vi "Select Model.vi"(10 "SHIFT":enum16{"1", "2", "3", "G"}(ring)) -> (1 "Cancelled":bool, 2 "Initial Data":T2)   [LabVIEW 2017]
uses:
  controls/Model Name.ctl
  GV/All Inputs.vi
panel:
  out "SACB Status":string
  in  "Cancel":bool
  out "Error Out":errorcluster
  out "Connected?":bool caption="Connected to SACB?"
  in  "Model Name":T1=enum."W 501 FRH Std."
  in  "OK Button":bool
  in  "ID":string
  # "Start Autocycle"
  # "Please select the model that you wish to run the autocyle test for, enter the operator ID and then click OK."
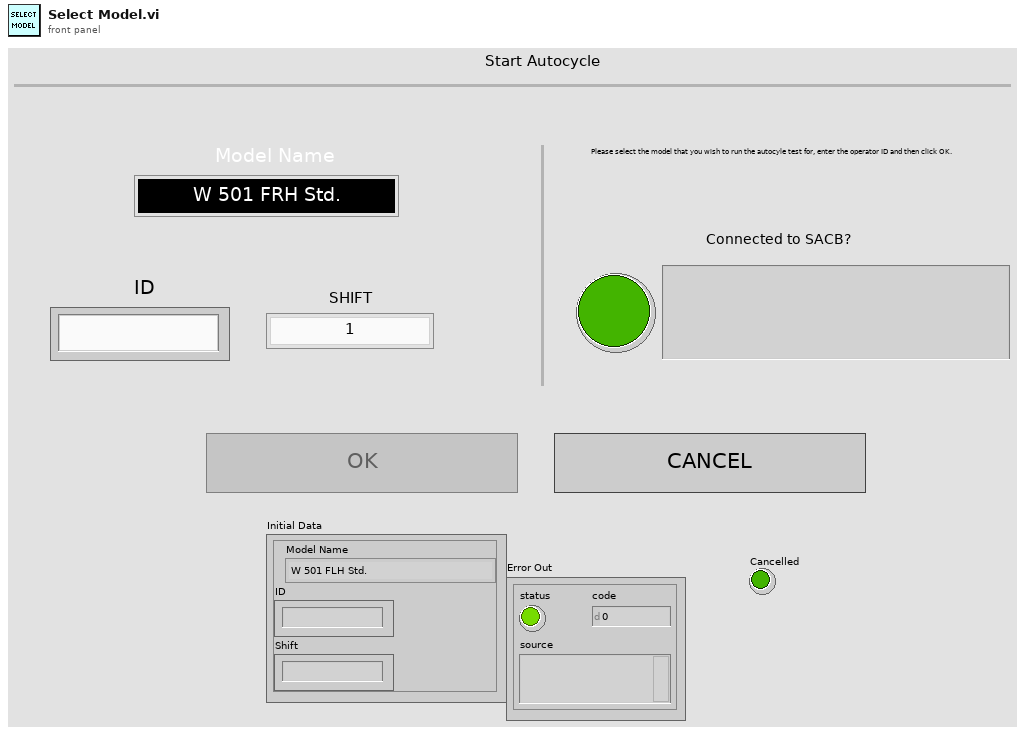
[diagram p1: front panel]
types:
  T1 = typedef "Model Name.ctl" = enum16{"W 501 FLH Std.", "W 501 FRH Std.", "W 601 FR RH Std", "W 601 FR LH Std", "W 601 RR RH Std", "W 601 RR LH Std", "W 601 FR RH AP", "W 601 FR LH AP", "W 601 RR RH AP", "W 601 RR LH AP"}
  T2 = cluster{"Model Name":T1, "ID":string, "Shift":string}
  T3 = enum8{"Enabled", "Disabled", "Disabled and Grayed Out"}
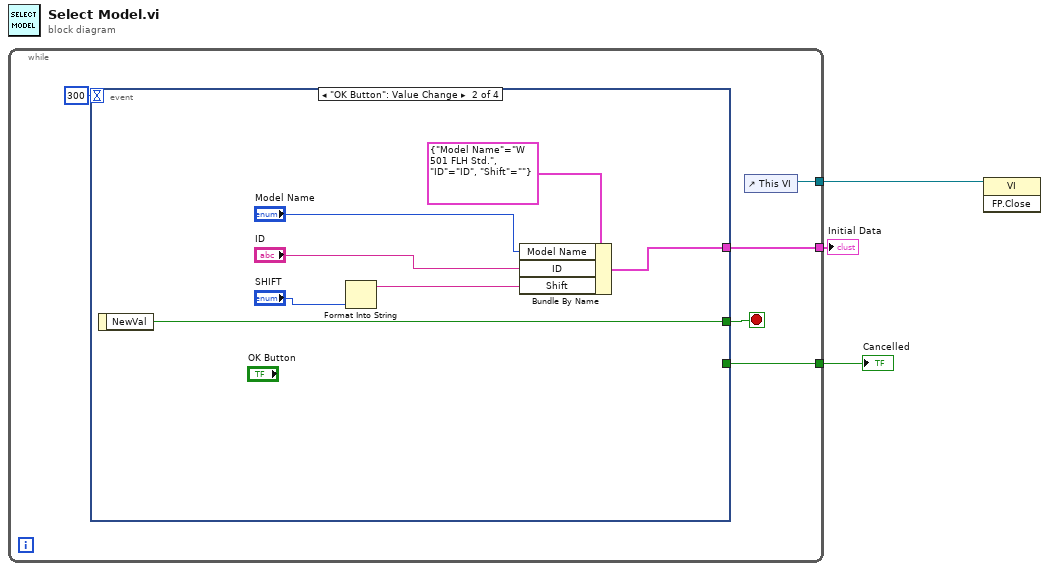
[diagram p0: block diagram]
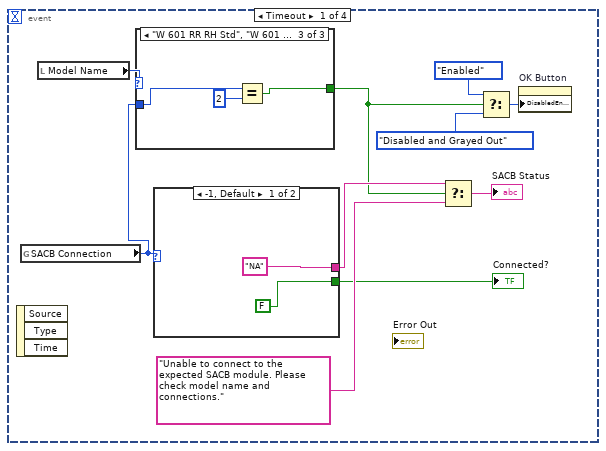
[diagram p2: hidden frame]
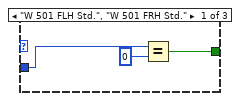
[diagram p3: hidden frame]
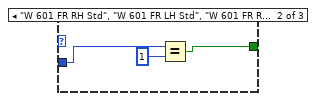
[diagram p4: hidden frame]
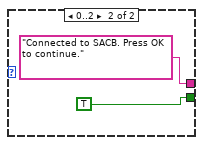
[diagram p5: hidden frame]
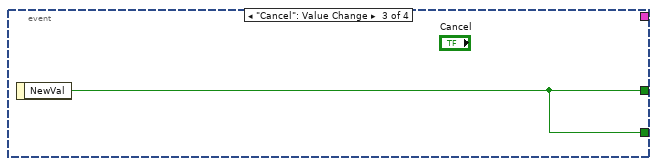
[diagram p6: hidden frame]
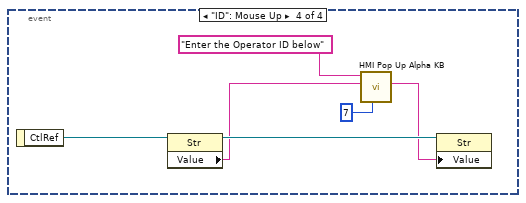
[diagram p7: hidden frame]
diagram:
  n1 = while {
    tunnel: [w8] -> w2
    tunnel: [w5] -> w3
    tunnel: [w4] -> w1
    stop <- w7 stop-if-true
    n2 = event shown="[1] \"OK Button\": Value Change" {
      selector: _ -> [_ _ _ _]
      dyn-events: _ -> [_ _ _ _]
      timeout: 300 -> [_ _ _ _]
      tunnel: [_ w36 _ _] -> w8
      tunnel: [_ w35 w39 _] -> w7
      tunnel: [_ _ w39 _] -> w5
      event Timeout {
        n3 = event-data() -> ()  [unwired: 1 in, 3 out]
        n4 = global read "All Inputs.vi" "SACB Connection"() -> (w10:i32)
        n5 = local read "Model Name"() -> (w11:T1)
        n6 = case shown="\"W 601 RR RH Std\", \"W 601 RR LH Std\", \"W 601 RR RH AP\", \"W 601 RR LH AP\"" w11 {
          tunnel: w10 -> [w21 w24 w27]
          tunnel: [w19 w22 w25] -> w9
          frame "W 501 FLH Std.", "W 501 FRH Std." {
            n7 = Equal?(x=w21, y=0) -> (x = y?=w19:bool)
          }
          frame "W 601 FR RH Std", "W 601 FR LH Std", "W 601 FR RH AP", "W 601 FR LH AP" {
            n8 = Equal?(x=w24, y=1) -> (x = y?=w22:bool)
          }
          frame "W 601 RR RH Std", "W 601 RR LH Std", "W 601 RR RH AP", "W 601 RR LH AP" {
            n9 = Equal?(x=w27, y=2) -> (x = y?=w25:bool)
          }
        }
        n10 = case shown="-1, Default" w10 {
          tunnel: ["NA" "Connected to SACB. Press OK to continue." ("SACB Status")] -> w13
          tunnel: [FALSE TRUE] -> w12
          frame -1, Default {
          }
          frame 0..2 {
          }
        }
        "Connected?" <- w12
        n11 = Select(t=w13, s=w9, f="Unable to connect to the expected SACB module. Please check model name and connections." ("SACB Status")) -> (s? t:f=→"SACB Status":string)
        n12 = Select(t=T3."Enabled" ("Disabled"), s=w9, f=T3."Disabled and Grayed Out" ("Disabled")) -> (s? t:f=w18:T3)
        n13 = property on="OK Button" class="Bool"("DisabledEnum"=w18) -> ()  [unwired: 2 in, 2 out]
      }
      event "OK Button": Value Change {
        n14 = event-data() -> ("NewVal"=w35:bool)  [unwired: 1 in]
        n15 = Format Into String("SHIFT") -> (resulting string=w33:string)  [unwired: 3 in, 1 out]
        n16 = Bundle By Name(cluster=T2 {"Model Name"=enum."W 501 FLH Std.", "ID"="ID", "Shift"=""} ("Initial Data"), "Model Name"="Model Name", "ID"="ID", "Shift"=w33) -> (w36:T2)
      }
      event "Cancel": Value Change {
        n17 = event-data() -> ("NewVal"=w39:bool)  [unwired: 1 in]
      }
      event "ID": Mouse Up {
        n18 = event-data() -> ("CtlRef"=w43:refnum<vi>)  [unwired: 1 in]
        n19 = property class="Str"(reference=w43) -> (reference out=w42:refnum<vi>, "Value"=w40:string)  [unwired: 1 in, 1 out]
        n20 = call "HMI Pop Up Alpha KB.vi"("Max Length (70)"=7, "String In"=w40, "Message In"="Enter the Operator ID below") -> ("String Out"=w41:string)  [unwired: 7 in, 1 out]
        n21 = property class="Str"(reference=w42, "Value"=w41) -> ()  [unwired: 1 in, 2 out]
      }
    }
    n22 = control-ref of="This VI"() -> (w4:refnum<vi>)
  }
  "Cancelled" <- w3
  "Initial Data" <- w2
  n23 = invoke class="VI" method="FP.Close"(reference=w1) -> ()  [unwired: 2 in, 3 out]
